vi "spec_get_cupconfiglist.vi"(8 "error in (no error)":errorcluster, 11 "Qtegra in":refnum<class "Qtegra.lvclass">) -> (0 "error out":errorcluster, 2 "CupConfigList":string, 3 "Qtegra out":refnum<class "Qtegra.lvclass">)   [LabVIEW 2017, in "Qtegra.lvclass"]
doc: "Get a list of all available CupConfiguration from the instrument.\nMainly applies to Qtegra"
uses:
  Qtegra.lvclass
  \\Mac\Home/my data/privat/Software/LabView/MSControlSuite_Code/MSControl/Classes/Instrument/instrument.lvclass
  global variables.vi
  instrument.lvclass
  StatusLog/StatusLog.lvclass
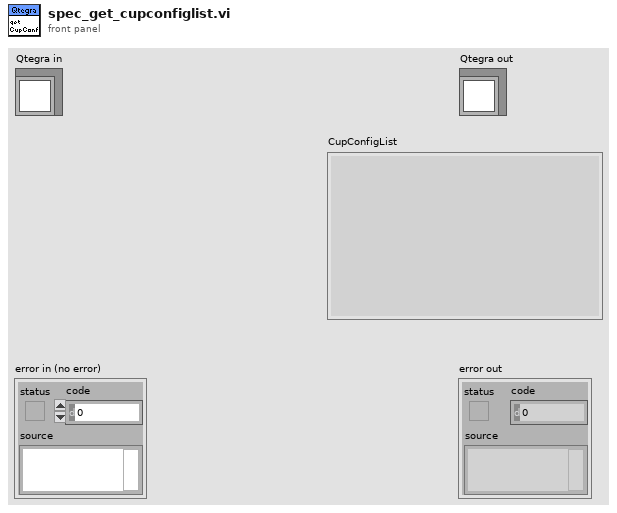
[diagram p1: front panel]
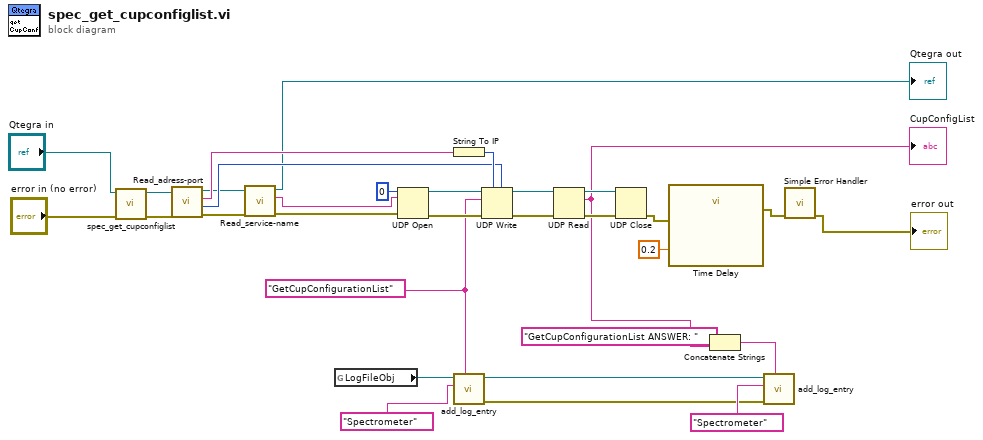
[diagram p0: block diagram]
diagram:
  w4 = "GetCupConfigurationList" ("format string")
  n1 = call-parent "spec_get_cupconfiglist.vi"("error in (no error)"="error in (no error)", "instrument in"="Qtegra in") -> ("error out"=w6:errorcluster, "instrument out"=w7:refnum<class "Qtegra.lvclass">)  [unwired: 7 in, 1 out]
  n2 = call "Read_adress-port.vi"("error in (no error)"=w6, "instrument in"=w7) -> ("error out"=w22:errorcluster, "port number"=w23:i32, "adress"=w30:string, "instrument out"=w21:refnum<class "Qtegra.lvclass">)  [unwired: 6 in]
  n3 = call-dynamic "Read_service-name.vi"("error in (no error)"=w22, "instrument in"=w21) -> ("error out"=w20:errorcluster, "service name"=w19:string, "instrument out"=→"Qtegra out":refnum<class "Qtegra.lvclass">)  [unwired: 7 in]
  n4 = global read "global variables.vi" "LogFileObj"() -> (w11:refnum<class "StatusLog.lvclass">)
  n5 = UDP Open(8:w20, 10:w19, 11:u16 0 ("port")) -> (port=w26:refnum<k16>, 0:w27:errorcluster)  [unwired: 2 in, 1 out]
  n6 = String To IP(1:w30) -> (0:w29:u32)
  n7 = call-dynamic "add_log_entry.vi"("new entry"=w4, "log identifiers"="Spectrometer", "StatusLog in"=w11) -> ("error out"=w8:errorcluster, "StatusLog out"=w10:refnum<class "StatusLog.lvclass">)  [unwired: 5 in]
  n8 = UDP Write(address=w29, port or service name=w23, connection ID=w26, data in=w4, 8:w27) -> (error out=w24:errorcluster, 3:w25:refnum<k16>)  [unwired: 1 in]
  n9 = UDP Read(connection ID=w25, 8:w24) -> (data out=w2:string, error out=w18:errorcluster, 3:w17:refnum<k16>)  [unwired: 2 in, 2 out]
  "CupConfigList" <- w2
  n10 = UDP Close(connection ID=w17, 8:w18) -> (error out=w16:errorcluster)  [unwired: 1 out]
  n11 = call "Time Delay"("error in (no error)"=w16, "Delay Time (s)"=0.2) -> ("error out"=w15:errorcluster)  [unwired: 9 in]
  n12 = Concatenate Strings("GetCupConfigurationList ANSWER: ", w2) -> (w3:string)
  n13 = call-dynamic "add_log_entry.vi"("new entry"=w3, "error in (no error)"=w8, "log identifiers"="Spectrometer", "StatusLog in"=w10) -> ()  [unwired: 4 in, 2 out]
  n14 = call <vilib>:"Simple Error Handler.vi"("error in (no error)"=w15) -> ("error out"=→"error out":errorcluster)  [unwired: 4 in, 4 out]
